vi "Read Header.vi"(0 "Image Data in":u8[](array[numeric])) -> (1 "Image Data out":u8[](array[numeric]), 3 "ImFileDirectOffs":u32, 4 "isTIFF":bool)   [LabVIEW 2018, in "TIFF File Reader.lvlib"]
doc: "Reads the header of a tiff file to determine the version number and the location of the image data in the file. Format determines whether the image file is coded LSB or MSB, although the rest of the routines only understand PC image data !"
uses:
  TIFF File Reader.lvlib
  Globals.vi
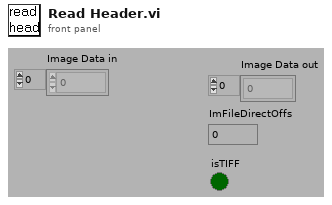
[diagram p1: front panel]
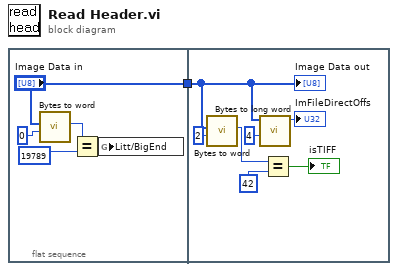
[diagram p0: block diagram]
diagram:
  n1 = flat-sequence {
    tunnel: ["Image Data in"] -> w1
    tunnel: w1 -> [w7]
    frame #0 {
      n2 = call "Bytes to word.vi"("Index"=0, "Image Data in"="Image Data in") -> ("Word"=w3:u16)  [unwired: 1 in, 6 out]
      n3 = Equal?(x=w3, y=u16 19789) -> (x = y?=w6:bool)
      n4 = global write "Globals.vi" "Litt/BigEnd"(w6) -> ()
    }
    frame #1 {
      n5 = call "Bytes to word.vi"("Index"=2, "Image Data in"=w7) -> ("Word"=w8:u16)  [unwired: 1 in, 6 out]
      n6 = call "Bytes to long word.vi"("Index"=4, "Image Data in"=w7) -> ("U32"=→"ImFileDirectOffs":u32)  [unwired: 7 out]
      n7 = Equal?(x=w8, y=u16 42 ("Word")) -> (x = y?=→"isTIFF":bool)
      "Image Data out" <- w7
    }
  }
